vi "myRIO_BRig_RT_dataBlock_BTPR__R.vi"() -> (2 "output_BTPR__R":i32)   [LabVIEW 2014]
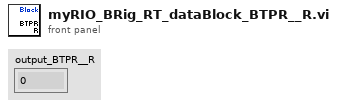
[diagram p1: front panel]
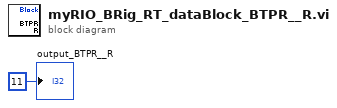
[diagram p0: block diagram]
diagram:
  "output_BTPR__R" <- 11 ("output_iBlock")
